vi "DAQ- Steper 1.vi"(2 "error in":errorcluster, 3 "Speed d/s":dbl=10.0, 4 "Mode":i32(ring)=10178 items=["Finite Samples"=10178, "Continuous Samples"=10123, "Hardware Timed Single Point"=12522], 5 "Travel (Degree)":dbl=100.0) -> (0 "error out":errorcluster, 1 "Task Done Bit":bool)   [LabVIEW 2015]
uses:
  <vilib>/DAQmx/create/channels.llb/DAQmx Create Channel (CO-Pulse Generation-Frequency).vi
  <vilib>/DAQmx/configure/timing.llb/DAQmx Timing (Implicit).vi
panel:
  out "32bit integer":i32
  in  "Motor PPR":dbl=36000.0
  in  "Motor Gear Ratio":dbl=1.0
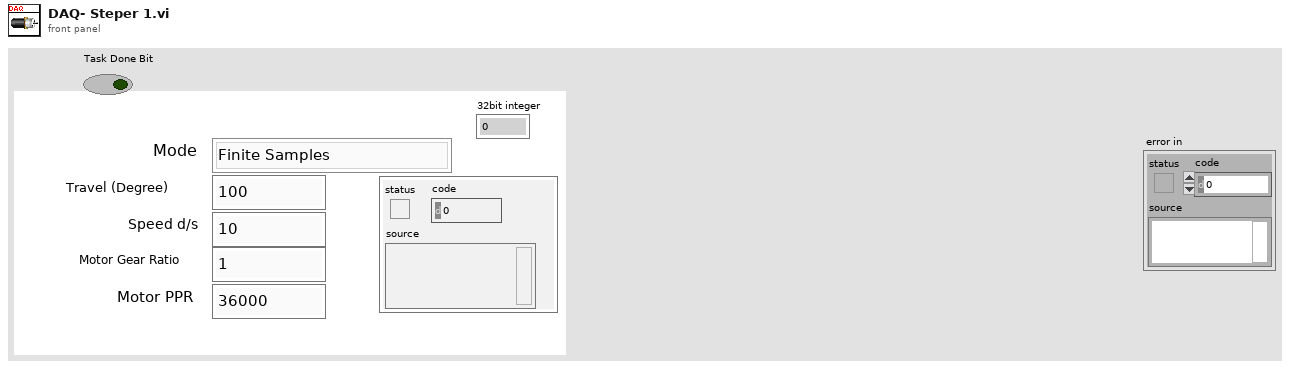
[diagram p1: front panel]
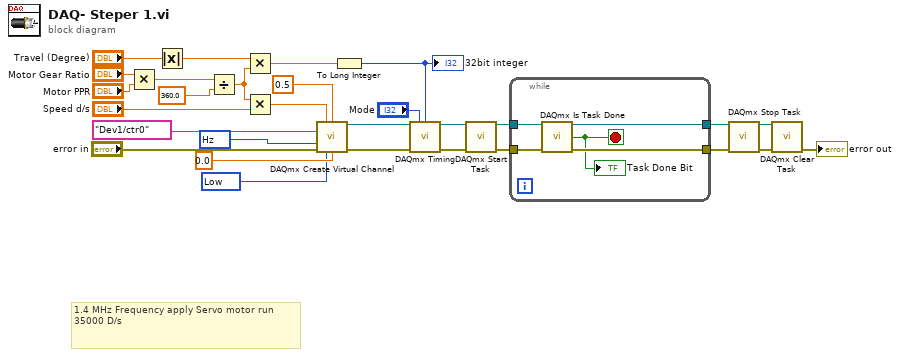
[diagram p0: block diagram]
diagram:
  w3 = 10373 items=["Hz"=10373] ("units")
  w4 = 10214 items=["High"=10192, "Low"=10214] ("idle state")
  # "1.4 MHz Frequency apply Servo motor run \n35000 D/s"
  n1 = Multiply(x="Motor Gear Ratio", y="Motor PPR") -> (x*y=w14:dbl)
  n2 = Absolute Value(x="Travel (Degree)") -> (abs(x)=w13:dbl)
  n3 = Divide(x=w14, y=360.0) -> (x/y=w20:dbl)
  n4 = Multiply(x=w13, y=w20) -> (x*y=w18:dbl)
  n5 = Multiply(x=w20, y="Speed d/s") -> (x*y=w26:dbl)
  n6 = call-poly <vilib>:"DAQmx Create Virtual Channel.vi"("frequency"=w26, "duty cycle"=0.5, "counter"=tag "Dev1/ctr0", "units"=w3, "error in"="error in", "idle state"=w4, "initial delay"=0.0) -> ("task out"=w6:refnum<k21>, "error out"=w7:errorcluster)  [unwired: 7 in]
  n7 = To Long Integer(number=w18) -> (32bit integer=w29:i32)
  "32bit integer" <- w29
  n8 = call-poly <vilib>:"DAQmx Timing.vi"("task/channels in"=w6, "sample mode"="Mode", "samples per channel"=w29, "error in"=w7) -> ("task out"=w8:refnum<k21>, "error out"=w9:errorcluster)  [unwired: 10 in]
  n9 = call <vilib>:"DAQmx Start Task.vi"("task/channels in"=w8, "error in"=w9) -> ("task out"=w1:refnum<k21>, "error out"=w2:errorcluster)  [unwired: 12 in]
  n10 = while {
    tunnel: w1 -> [w34]
    tunnel: [w33] -> w10
    tunnel: w2 -> [w31]
    tunnel: [w32] -> w24
    stop <- w30 stop-if-true
    n11 = call <vilib>:"DAQmx Is Task Done.vi"("task/channels in"=w34, "error in"=w31) -> ("task out"=w33:refnum<k21>, "task done?"=w30:bool, "error out"=w32:errorcluster)  [unwired: 11 in]
    "Task Done Bit" <- w30
  }
  n12 = call <vilib>:"DAQmx Stop Task.vi"("task/channels in"=w10, "error in"=w24) -> ("task out"=w11:refnum<k21>, "error out"=w25:errorcluster)  [unwired: 12 in]
  n13 = call <vilib>:"DAQmx Clear Task.vi"("task in"=w11, "error in"=w25) -> ("error out"=→"error out":errorcluster)  [unwired: 13 in]
